vi "Actor Main Run VI Name.vi"() -> (0 "Actor Main Run VI Name":string)   [LabVIEW 2018, in "Scripting.lvlib"]
uses:
  Scripting.lvlib
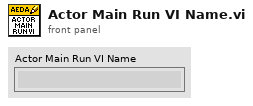
[diagram p1: front panel]
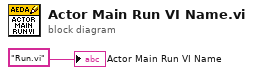
[diagram p0: block diagram]
diagram:
  "Actor Main Run VI Name" <- "Run.vi" ("y")
